vi "Get position of Param Name and Value from 1D array.vi"(11 "1D path array":string[](array[string])) -> (2 "Index of Param Value":i32, 3 "Index of Param Name":i32)   [LabVIEW 2012]
doc: "SciScan 1.2 160622"
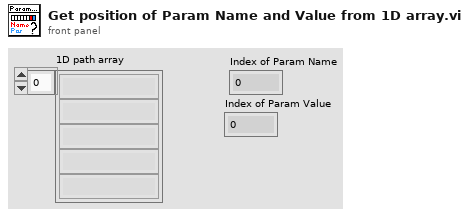
[diagram p1: front panel]
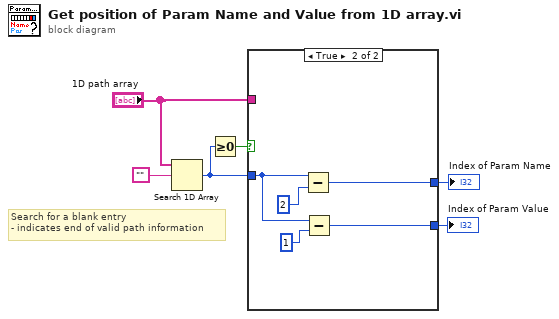
[diagram p0: block diagram]
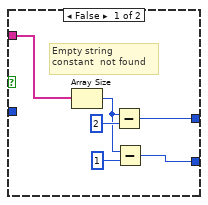
[diagram p2: hidden frame]
diagram:
  # "Search for a blank entry\n- indicates end of valid path information"
  n1 = Search 1D Array(1D array="1D path array", element="") -> (index of element=w4:i32)  [unwired: 1 in]
  n2 = Greater Or Equal To 0?(x=w4) -> (x >= 0?=w5:bool)
  n3 = case shown="True" w5 {
    tunnel: w4 -> [_ w14]
    tunnel: "1D path array" -> [w12 _]
    tunnel: [w10 w16] -> w3
    tunnel: [w7 w13] -> w1
    frame False {
      # "Empty string\nconstant  not found"
      n4 = Array Size(array=w12) -> (size(s)=w9:i32)
      n5 = Subtract(x=w9, y=2) -> (x-y=w10:i32)
      n6 = Subtract(x=w9, y=1) -> (x-y=w7:i32)
    }
    frame True {
      n7 = Subtract(x=w14, y=2) -> (x-y=w16:i32)
      n8 = Subtract(x=w14, y=1) -> (x-y=w13:i32)
    }
  }
  "Index of Param Name" <- w3
  "Index of Param Value" <- w1
